vi "Tester.vi"() -> ()   [LabVIEW 2018]
uses:
  <vilib>/NI/Modbus Library/API/Modbus API.lvclass/Modbus API.ctl
  <vilib>/NI/Modbus Library/Transmission Data Unit/Transmission Data Unit.lvclass/Transmission Data Unit.ctl
  <vilib>/NI/Modbus Library/Transmission Data Unit/Write Unit ID.vi
  <vilib>/NI/Modbus Library/API/Read Transmission Data Unit.vi
  <vilib>/NI/Modbus Library/API/Write Transmission Data Unit.vi
  <vilib>/NI/Modbus Library/API/Master/Modbus Master.lvclass
  C:/Program Files (x86)/National Instruments/LabVIEW 2018/vi.lib/NI/Modbus Library/API/Modbus API.lvclass
  <vilib>/NI/Modbus Library/API/Wrapper/Create Serial Master.vi
  <vilib>/NI/Modbus Library/API/Wrapper/API Main.lvlib
panel:
  in  "OK Button":bool
  in  "register to write":u16
  in  "stop":bool
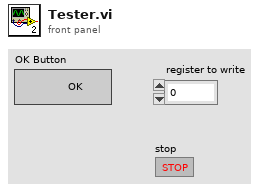
[diagram p1: front panel]
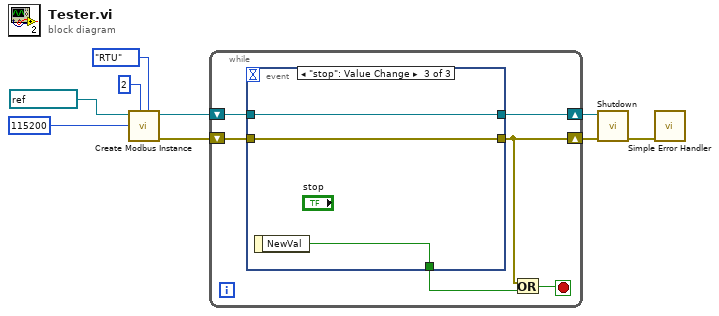
[diagram p0: block diagram]
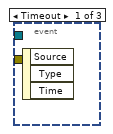
[diagram p2: hidden frame]
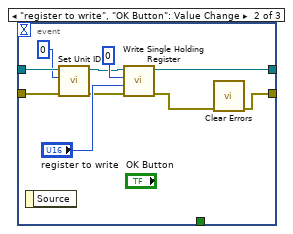
[diagram p3: hidden frame]
diagram:
  n1 = call-poly <vilib>:"Create Modbus Instance.vi"("serial type"=enum16{"RTU", "ASCII"}."RTU", "unit ID"=u8 2, "baud rate"=u32 115200, "VISA resource name"=refnum<visa-resource-name> "COM16") -> ("error out"=w4:errorcluster, "serial master instance"=w5:refnum<class "Modbus Master.lvclass">)  [unwired: 6 in]
  n2 = while {
    shift-right: [w13] -> w3
    shift-left: w5 -> [w15]
    shift-right: [w12] -> w2
    shift-left: w4 -> [w14]
    stop <- w10 stop-if-true
    n3 = event shown="[2] \"stop\": Value Change" {
      selector: _ -> [_ _ _]
      dyn-events: _ -> [_ _ _]
      timeout: _ -> [_ _ _]
      tunnel: [_ _ w26] -> w11
      tunnel: w15 -> [_ w18 w27]
      tunnel: w14 -> [_ w23 w28]
      tunnel: [_ w22 w27] -> w13
      tunnel: [_ w20 w28] -> w12
      event Timeout {
        n4 = event-data() -> ()  [unwired: 1 in, 3 out]
      }
      event "register to write", "OK Button": Value Change {
        n5 = event-data() -> ()  [unwired: 1 in, 1 out]
        n6 = call <vilib>:"Set Unit ID.vi"("error in"=w23, "unit ID"=u8 0, "Modbus master in"=w18) -> ("error out"=w19:errorcluster, "Modbus master out"=w17:refnum<class "Modbus Master.lvclass">)  [unwired: 7 in]
        n7 = call-dynamic "Write Single Holding Register.vi"("error in"=w19, "register to write"="register to write", "address"=u16 0, "Modbus master in"=w17) -> ("error out"=w21:errorcluster, "Modbus master out"=w22:refnum<class "Modbus Master.lvclass">)  [unwired: 6 in]
        n8 = call <vilib>:"Clear Errors.vi"("error in (no error)"=w21) -> ("error out"=w20:errorcluster)  [unwired: 5 in, 1 out]
      }
      event "stop": Value Change {
        n9 = event-data() -> ("NewVal"=w26:bool)  [unwired: 1 in]
      }
    }
    n10 = Or(x=w12, y=w11) -> (x .or. y?=w10:bool)
  }
  n11 = call-dynamic "Shutdown.vi"("error in"=w2, "Modbus master in"=w3) -> ("error out"=w1:errorcluster)  [unwired: 9 in]
  n12 = call <vilib>:"Simple Error Handler.vi"("error in (no error)"=w1) -> ()  [unwired: 4 in, 5 out]
